vi "Stop Core.vi"(10 "final error code":i32, 11 "CI Mediator in":refnum<class "CI Mediator.lvclass">) -> (3 "CI Mediator out":refnum<class "CI Mediator.lvclass">)   [LabVIEW 2014, in "CI Mediator.lvlib" / "CI Mediator.lvclass"]
doc: "(<B>Filename</B>: Actor Framework.lvlib:Actor.lvclass:Stop Core.vi)\n\nDefines what the actor does before it stops. Use the <B>final error code</B> input to determine whether the actor shut down in response to an error.\n\nBy default, this method does nothing. A descendant class may override it to define behavior, such as shutting down any processes the actor initiated in its override of the Actor Core method."
uses:
  CI Mediator.lvclass
  CI Mediator.lvclass/CI Mediator.ctl
  <vilib>/ActorFramework/Actor/Actor.lvclass
  Classes/Executor/Executor.lvclass
  Classes/Log File/Log File.lvclass
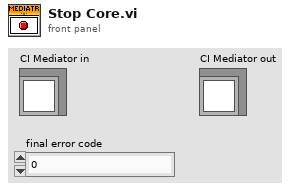
[diagram p1: front panel]
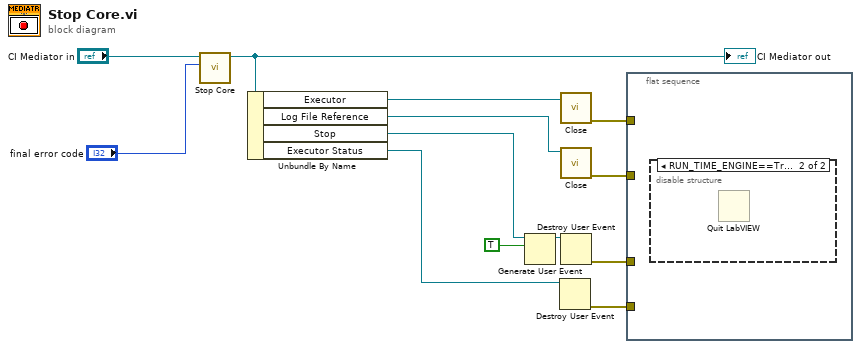
[diagram p0: block diagram]
diagram:
  n1 = call-parent "Stop Core.vi"("final error code"="final error code", "Actor in"="CI Mediator in") -> ("Actor out"=w11:refnum<class "CI Mediator.lvclass">)  [unwired: 9 in]
  "CI Mediator out" <- w11
  n2 = Unbundle By Name(w11) -> ("Executor"=w10:refnum<class "Executor.lvclass">, "Log File Reference"=w9:refnum<data-value>, "Stop"=w8:refnum<user-event>, "Executor Status"=w7:refnum<user-event>)
  n3 = Generate User Event(user event=w8, event data cluster=TRUE ("event data")) -> (user event out=w2:refnum<user-event>)  [unwired: 2 in, 1 out]
  n4 = Destroy User Event(user event=w7) -> (error out=w3:errorcluster)  [unwired: 1 in]
  n5 = call "Close.vi"("Executor"=w10) -> ("error out"=w6:errorcluster)  [unwired: 10 in]
  n6 = call "Close.vi"("Log File Ref"=w9) -> ("error out"=w5:errorcluster)  [unwired: 10 in]
  n7 = Destroy User Event(user event=w2) -> (error out=w4:errorcluster)  [unwired: 1 in]
  n8 = flat-sequence {
    tunnel: w6 -> [_]
    tunnel: w5 -> [_]
    tunnel: w4 -> [_]
    tunnel: w3 -> [_]
    frame #0 {
      n9 = disable-structure shown="RUN_TIME_ENGINE==True" {
        frame condition #0 (active) {
        }
        frame condition #1 {
          n10 = Quit LabVIEW() -> ()  [unwired: 1 in]
        }
      }
    }
  }
